vi "Start Data Pulse.vi"(8 "error in (no error)":errorcluster, 11 "3300 in":refnum<class "3300.lvclass">) -> (0 "error out":errorcluster, 3 "3300 out":refnum<class "3300.lvclass">)   [LabVIEW 2019, in "3300.lvlib" / "3300.lvclass"]
uses:
  Library/3300.lvclass
  C:/Users/Public/Documents/Development/builds/Instruments/Electronic Load.lvlibp/Library/Electronic Load.lvclass
  builds/Instruments/Electronic Load.lvlibp/Accessors/Trigger/Read All Pulse.vi
  builds/Instruments/Electronic Load.lvlibp/Accessors/Trigger/Read Pulse Enable.vi
  builds/Instruments/Electronic Load.lvlibp/Accessors/Read Available Channels.vi
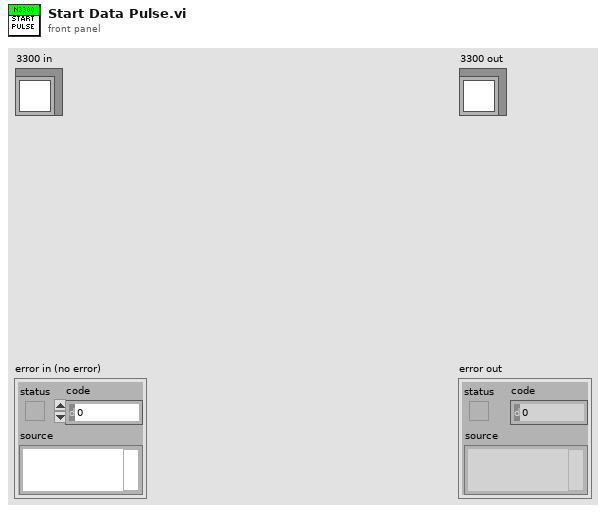
[diagram p1: front panel]
types:
  T1 = typedef "Electronic Load.lvlibp/Electronic Load.lvclass/Trigger Settings.ctl" = cluster{"Mode":T2, "Initial":dbl, "Transient":dbl, "Interval":dbl, "Width":dbl, "Delay":dbl, "Data Pts":i32, "Slew Rate":dbl}
  T2 = typedef "Electronic Load.lvlibp/Electronic Load.lvclass/E-Load Mode.ctl" = enum16{"Current", "Resistance", "Voltage"}
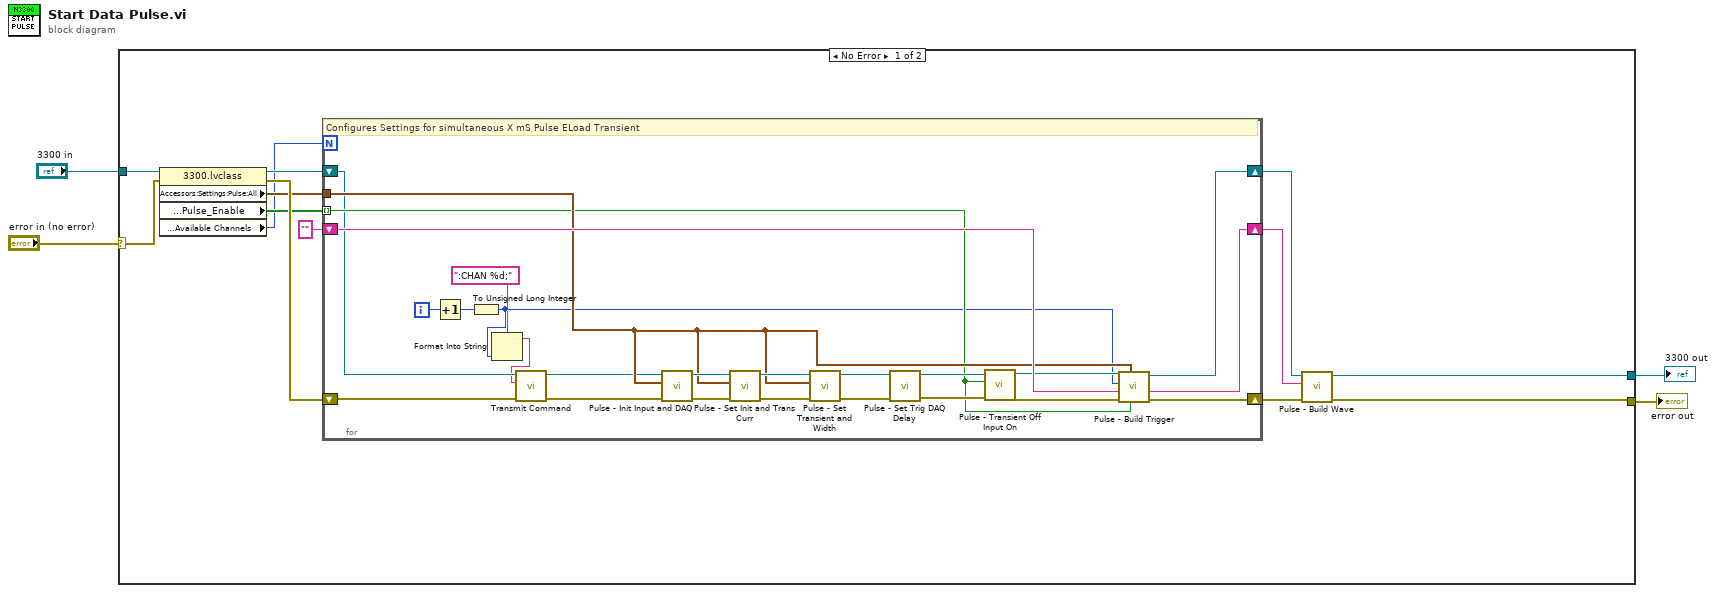
[diagram p0: block diagram]
diagram:
  n1 = case shown="No Error" "error in (no error)" {
    selector: "error in (no error)" -> [w14 w44]
    tunnel: [w8 w44] -> w3
    tunnel: [w9 w43] -> w1
    tunnel: "3300 in" -> [w16 w43]
    frame No Error {
      n2 = property class="3300.lvclass"(reference=w16, error in=w14) -> (reference out=w15:refnum<class "3300.lvclass">, error out=w13:errorcluster, "Accessors:Settings:Pulse:All"=w7:T1, "Accessors:Settings:Pulse:Pulse_Enable"=w6:bool[], "Accessors:Configuration:Available Channels"=w5:i32)
      n3 = for {
        N: w5 -> [_]
        shift-right: [w40] -> w12
        shift-left: w13 -> [w23]
        shift-right: [w41] -> w10
        shift-left: "" -> [w42]
        tunnel: w7 -> [w26]
        shift-right: [w39] -> w11
        shift-left: w15 -> [w24]
        tunnel: w6 -> [w25] mode=indexing
        i -> [w27]
        # "Configures Settings for simultaneous X mS Pulse ELoad Transient"
        n4 = Increment(x=w27) -> (x+1=w34:i32)
        n5 = To Unsigned Long Integer(number=w34) -> (unsigned 32bit integer=w20:u32)
        n6 = Format Into String(format string=":CHAN %d;", w20) -> (resulting string=w18:string)  [unwired: 2 in, 1 out]
        n7 = call "Transmit Command.vi"("error in"=w23, "Command"=w18, "3300 in"=w24) -> ("error out"=w22:errorcluster, "3300 out"=w21:refnum<class "3300.lvclass">)  [unwired: 7 in]
        n8 = call "Pulse - Init Input and DAQ.vi"("error in"=w22, "Trigger Settings"=w26, "3300 in"=w21) -> ("error out"=w30:errorcluster, "3300 out"=w33:refnum<class "3300.lvclass">)  [unwired: 7 in]
        n9 = call "Pulse - Set Init and Trans Curr.vi"("error in (no error)"=w30, "Trigger Settings"=w26, "3300 in"=w33) -> ("error out"=w29:errorcluster, "3300 out"=w32:refnum<class "3300.lvclass">)  [unwired: 7 in]
        n10 = call "Pulse - Set Transient and Width.vi"("error in (no error)"=w29, "Trigger Settings"=w26, "3300 in"=w32) -> ("error out"=w28:errorcluster, "3300 out"=w31:refnum<class "3300.lvclass">)  [unwired: 7 in]
        n11 = call "Pulse - Set Trig DAQ Delay.vi"("error in (no error)"=w28, "3300 in"=w31) -> ("error out"=w36:errorcluster, "3300 out"=w35:refnum<class "3300.lvclass">)  [unwired: 8 in]
        n12 = call "Pulse - Transient Off Input On.vi"("error in (no error)"=w36, "Trig Enable"=w25, "3300 in"=w35) -> ("error out"=w37:errorcluster, "3300 out"=w38:refnum<class "3300.lvclass">)  [unwired: 7 in]
        n13 = call "Pulse - Build Trigger.vi"("Enabled"=w25, "Trigger Settings"=w26, "error in (no error)"=w37, "Single Command In"=w42, "Channel (1)"=w20, "3300 in"=w38) -> ("error out"=w40:errorcluster, "Single Command Out"=w41:string, "3300 out"=w39:refnum<class "3300.lvclass">)  [unwired: 3 in]
      }
      n14 = call "Pulse - Build Wave.vi"("error in (no error)"=w12, "Channel List String"=w10, "3300 in"=w11) -> ("error out"=w8:errorcluster, "3300 out"=w9:refnum<class "3300.lvclass">)  [unwired: 7 in]
    }
    frame Error {
    }
  }
  "error out" <- w3
  "3300 out" <- w1
